vi "TelemetryFieldToAddress.vi"(11 "TelemetryFields":T1=enum."AnalogInputRaw4") -> (3 "Address":u32)   [LabVIEW 2018]
uses:
  TelemetryFields.ctl
  <vilib>/Platform/TimedLoop/XDataNode/timing_clust.ctl
  <vilib>/Platform/TimedLoop/XDataNode/nitl_modes.ctl
  <vilib>/Platform/TimedLoop/XDataNode/wakeup.ctl
  <vilib>/rvi/Emulation/niFpgaSctlEmulationGetInTimedLoop.vi
  <vilib>/rvi/Emulation/niFpgaEmulationReportErrorSimple.vi
  <vilib>/rvi/Emulation/niFpgaGetClockAttributes.vi
  <vilib>/rvi/Emulation/niFpgaCriticalErrorInLSC.vi
  <vilib>/Platform/TimedLoop/XDataNode/XDataNode.xnode
  <vilib>/Platform/TimedLoop/XDataNode/XDNodeRunTimeDep.lvlib
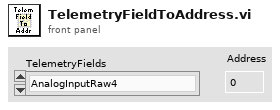
[diagram p1: front panel]
types:
  T1 = typedef "TelemetryFields.ctl" = enum16{"None", "AnalogInputSampleCount", "AnalogInputSampleTimestamp", "AnalogInputRaw1", "AnalogInputRaw2", "AnalogInputRaw3", "AnalogInputRaw4", "AnalogInputRaw5", "AnalogInputRaw6", "AnalogInputRaw7", "AnalogInputRaw8", "AnalogInputRaw9", "AnalogInputRaw10", "AnalogInputRaw11", "AnalogInputRaw12", "AnalogInputRaw13", "AnalogInputRaw14", "AnalogInputRaw15", "AnalogInputRaw16", "DigitalInputSampleCount", "DigitalInputSampleTimestamp", "DigitalInputStates", "ThermocoupleSampleCount", "ThermocoupleSampleTimestamp", "ThermocoupleRaw1", "ThermocoupleRaw2", "ThermocoupleRaw3", "ThermocoupleRaw4", "ThermocoupleRaw5", "ThermocoupleRaw6", "ThermocoupleRaw7", "ThermocoupleRaw8", "ThermocoupleRaw9", "ThermocoupleRaw10", "ThermocoupleRaw11", "ThermocoupleRaw12", "ThermocoupleRaw13", "ThermocoupleRaw14", "ThermocoupleRaw15", "ThermocoupleRaw16", "WindSensorTxBytes", "WindSensorTxFrames", "WindSensorRxBytes", "WindSensorRxFrames", "WindSensorErrorTimestamp", "WindSensorErrorCode", "WindSensorSampleTimestamp", "WindSensorXRaw", "WindSensorYRaw", "WindSensorZRaw", "WindSensorSonicTempRaw", "WindSensorDiagWord", "WindSensorRecordCount", "FlowSensorTxBytes", "FlowSensorTxFrames", "FlowSensorRxBytes", "FlowSensorRxFrames", "FlowSensorErrorTimestamp", "FlowSensorErrorCode", "FlowSensorSampleTimestamp", "FlowSensorSignalStrength", "FlowSensorFlowRate", "FlowSensorNetTotalizer", "FlowSensorPositiveTotalizer", "FlowSensorNegativeTotalizer", "FlowSensorTemperature1", "FlowSensorTemperature2", "VFDTxBytes", "VFDTxFrames", "VFDRxBytes", "VFDRxFrames", "VFDErrorTimestamp", "VFDErrorCode", "VFDSampleTimestamp", "VFDVelocityBits", "VFDDiagnosticCode", "VFDFrequencyCommand", "VFDOutputFrequency", "VFDOutputCurrent", "VFDDCBusVoltage", "VFDOutputVoltage"}
  T2 = typedef "XDNodeRunTimeDep.lvlib/timing_clust.ctl" = cluster{"Expected End [f-1]":u64, "Actual End [f-1]":u64, "Finished Late? [f-1]":bool, "Expected End [i-1]":u64, "Actual End [i-1]":u64, "Finished Late? [i-1]":bool, "Expected Start [i]":u64, "Actual Start [i]":u64, "Expected Start [f]":u64, "Actual Start [f]":u64, "Source Name":string, "Structure Name":string, "Period":i64, "Deadline":i64, "Offset":i64, "Start":i64, "Priority":i32, "Timeout":i32, "Mode":T3, "Wakeup Reason":T4, "Error":errorcluster, "Source Type":string, "Secondary Source Type":string, "Global End Time":u64, "Global Start Time":u64, "Frame Duration":u64, "Iteration Duration":u64, "Assigned CPU":i32, "I/O Scan Engine Mode":u32}
  T3 = typedef "XDNodeRunTimeDep.lvlib/nitl_modes.ctl" = enum32{"No Change", "Process missed periods, maintain original phase", "Discard missed periods, maintain original phase", "Process missed periods, ignore original phase", "Discard missed periods, ignore original phase"}
  T4 = typedef "XDNodeRunTimeDep.lvlib/wakeup.ctl" = enum32{"Normal", "Aborted", "Asynchronous wakeup", "Timing source error", "Timed loop error", "Timeout"}
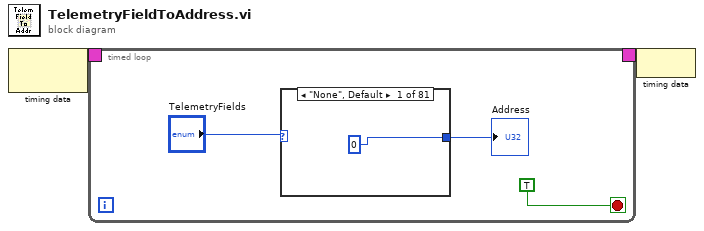
[diagram p0: block diagram]
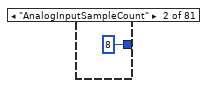
[diagram p2: hidden frame]
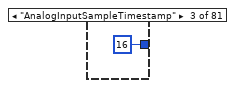
[diagram p3: hidden frame]
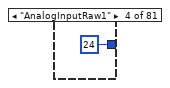
[diagram p4: hidden frame]
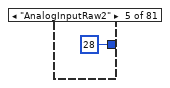
[diagram p5: hidden frame]
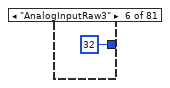
[diagram p6: hidden frame]
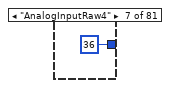
[diagram p7: hidden frame]
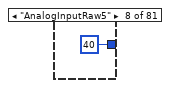
[diagram p8: hidden frame]
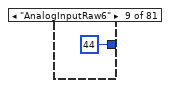
[diagram p9: hidden frame]
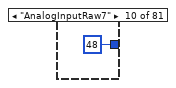
[diagram p10: hidden frame]
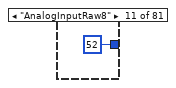
[diagram p11: hidden frame]
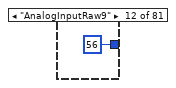
[diagram p12: hidden frame]
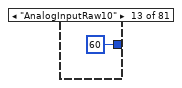
[diagram p13: hidden frame]
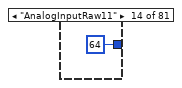
[diagram p14: hidden frame]
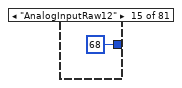
[diagram p15: hidden frame]
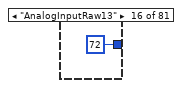
[diagram p16: hidden frame]
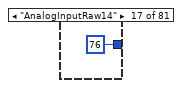
[diagram p17: hidden frame]
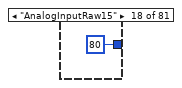
[diagram p18: hidden frame]
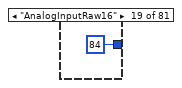
[diagram p19: hidden frame]
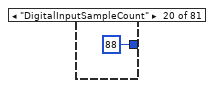
[diagram p20: hidden frame]
diagram:
  n1 = node-c288() -> (w2:T2)  [unwired: 1 in]
  n2 = timed-loop {
    timing: w2 -> [_]
    timing-out: [_] -> w1
    stop <- TRUE stop-if-true
    n3 = case shown="\"None\", Default" "TelemetryFields" {
      tunnel: [u32 0 ("Address") u32 8 ("Address") u32 16 ("Address") u32 24 ("Address") u32 28 ("Address") u32 32 ("Address") u32 36 ("Address") u32 40 ("Address") u32 44 ("Address") u32 48 ("Address") u32 52 ("Address") u32 56 ("Address") u32 60 ("Address") u32 64 ("Address") u32 68 ("Address") u32 72 ("Address") u32 76 ("Address") u32 80 ("Address") u32 84 ("Address") u32 88 ("Address") u32 96 ("Address") u32 104 ("Address") u32 108 ("Address") u32 116 ("Address") u32 124 ("Address") u32 128 ("Address") u32 132 ("Address") u32 136 ("Address") u32 140 ("Address") u32 144 ("Address") u32 148 ("Address") u32 152 ("Address") u32 156 ("Address") u32 160 ("Address") u32 164 ("Address") u32 168 ("Address") u32 172 ("Address") u32 176 ("Address") u32 180 ("Address") u32 184 ("Address") u32 188 ("Address") u32 196 ("Address") u32 204 ("Address") u32 212 ("Address") u32 220 ("Address") u32 228 ("Address") u32 229 ("Address") u32 237 ("Address") u32 241 ("Address") u32 245 ("Address") u32 249 ("Address") u32 253 ("Address") u32 255 ("Address") u32 256 ("Address") u32 264 ("Address") u32 272 ("Address") u32 280 ("Address") u32 288 ("Address") u32 296 ("Address") u32 297 ("Address") u32 305 ("Address") u32 309 ("Address") u32 313 ("Address") u32 317 ("Address") u32 321 ("Address") u32 325 ("Address") u32 329 ("Address") u32 333 ("Address") u32 341 ("Address") u32 349 ("Address") u32 357 ("Address") u32 365 ("Address") u32 373 ("Address") u32 374 ("Address") u32 382 ("Address") u32 384 ("Address") u32 386 ("Address") u32 388 ("Address") u32 390 ("Address") u32 392 ("Address") u32 394 ("Address")] -> w3
      frame "None", Default {
      }
      frame "AnalogInputSampleCount" {
      }
      frame "AnalogInputSampleTimestamp" {
      }
      frame "AnalogInputRaw1" {
      }
      frame "AnalogInputRaw2" {
      }
      frame "AnalogInputRaw3" {
      }
      frame "AnalogInputRaw4" {
      }
      frame "AnalogInputRaw5" {
      }
      frame "AnalogInputRaw6" {
      }
      frame "AnalogInputRaw7" {
      }
      frame "AnalogInputRaw8" {
      }
      frame "AnalogInputRaw9" {
      }
      frame "AnalogInputRaw10" {
      }
      frame "AnalogInputRaw11" {
      }
      frame "AnalogInputRaw12" {
      }
      frame "AnalogInputRaw13" {
      }
      frame "AnalogInputRaw14" {
      }
      frame "AnalogInputRaw15" {
      }
      frame "AnalogInputRaw16" {
      }
      frame "DigitalInputSampleCount" {
      }
      frame "DigitalInputSampleTimestamp" {
      }
      frame "DigitalInputStates" {
      }
      frame "ThermocoupleSampleCount" {
      }
      frame "ThermocoupleSampleTimestamp" {
      }
      frame "ThermocoupleRaw1" {
      }
      frame "ThermocoupleRaw2" {
      }
      frame "ThermocoupleRaw3" {
      }
      frame "ThermocoupleRaw4" {
      }
      frame "ThermocoupleRaw5" {
      }
      frame "ThermocoupleRaw6" {
      }
      frame "ThermocoupleRaw7" {
      }
      frame "ThermocoupleRaw8" {
      }
      frame "ThermocoupleRaw9" {
      }
      frame "ThermocoupleRaw10" {
      }
      frame "ThermocoupleRaw11" {
      }
      frame "ThermocoupleRaw12" {
      }
      frame "ThermocoupleRaw13" {
      }
      frame "ThermocoupleRaw14" {
      }
      frame "ThermocoupleRaw15" {
      }
      frame "ThermocoupleRaw16" {
      }
      frame "WindSensorTxBytes" {
      }
      frame "WindSensorTxFrames" {
      }
      frame "WindSensorRxBytes" {
      }
      frame "WindSensorRxFrames" {
      }
      frame "WindSensorErrorTimestamp" {
      }
      frame "WindSensorErrorCode" {
      }
      frame "WindSensorSampleTimestamp" {
      }
      frame "WindSensorXRaw" {
      }
      frame "WindSensorYRaw" {
      }
      frame "WindSensorZRaw" {
      }
      frame "WindSensorSonicTempRaw" {
      }
      frame "WindSensorDiagWord" {
      }
      frame "WindSensorRecordCount" {
      }
      frame "FlowSensorTxBytes" {
      }
      frame "FlowSensorTxFrames" {
      }
      frame "FlowSensorRxBytes" {
      }
      frame "FlowSensorRxFrames" {
      }
      frame "FlowSensorErrorTimestamp" {
      }
      frame "FlowSensorErrorCode" {
      }
      frame "FlowSensorSampleTimestamp" {
      }
      frame "FlowSensorSignalStrength" {
      }
      frame "FlowSensorFlowRate" {
      }
      frame "FlowSensorNetTotalizer" {
      }
      frame "FlowSensorPositiveTotalizer" {
      }
      frame "FlowSensorNegativeTotalizer" {
      }
      frame "FlowSensorTemperature1" {
      }
      frame "FlowSensorTemperature2" {
      }
      frame "VFDTxBytes" {
      }
      frame "VFDTxFrames" {
      }
      frame "VFDRxBytes" {
      }
      frame "VFDRxFrames" {
      }
      frame "VFDErrorTimestamp" {
      }
      frame "VFDErrorCode" {
      }
      frame "VFDSampleTimestamp" {
      }
      frame "VFDVelocityBits" {
      }
      frame "VFDDiagnosticCode" {
      }
      frame "VFDFrequencyCommand" {
      }
      frame "VFDOutputFrequency" {
      }
      frame "VFDOutputCurrent" {
      }
      frame "VFDDCBusVoltage" {
      }
      frame "VFDOutputVoltage" {
      }
    }
    "Address" <- w3
  }
  n4 = node-c288(w1) -> ()
